vi "ge_TableFGV.vi"(4 "VKey":T1, 5 "Mod":bool, 6 "CtlRef":refnum<vi>, 7 "ge_TableCmnds":T7, 8 "error in":errorcluster, 9 "Cell Contents":T5, 10 "Specific Info":T4, 11 "ChanGrp.lvclass":refnum<class "ChanGrp.lvclass">) -> (0 "error out":errorcluster, 1 "Discard?":bool, 2 "ValIfDismissed":u16, 3 "ChanGrp.lvclass":refnum<class "ChanGrp.lvclass">)   [LabVIEW 2012]
uses:
  Custom Ctls Table/ge_TableCmnds.ctl
  Classes/Cfg Grandmaster/Class Chan Group/ChanGrp.lvclass
  Custom Ctls Table/ge_CellContents.ctl
  <vilib>/Utility/miscctls.llb/LVPoint32TypeDef.ctl
  Custom Ctls Table/ge_GrpSpecificInfo.ctl
  Common/Controls/TE_Designator.ctl
  <vilib>/event_ctls.llb/eventvkey.ctl
  Custom Ctrls/ge_FPCtrlRefLabel.ctl
  <vilib>/Utility/miscctls.llb/LVRowAndColumnTypeDef.ctl
  Custom Ctls Table/ge_StringVals.ctl
  Custom Ctls Table/ge_GlblCtrls.ctl
  <vilib>/Utility/miscctls.llb/LVRowAndColumnUnsignedTypeDef.ctl
  Custom Ctls Table/ge_HdrInfo.ctl
  Classes/Cfg Grandmaster/Class Chan Group/Read GrpName.vi
  Classes/Cfg Grandmaster/Class Chan Group/Read MeasType.vi
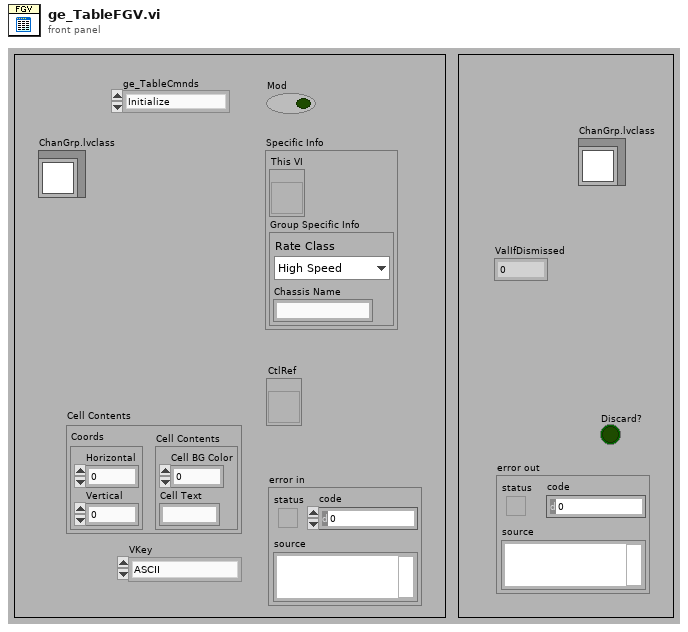
[diagram p1: front panel]
types:
  T1 = typedef "eventvkey.ctl" = enum16{"ASCII", "Enter", "Return", "Shift", "Ctrl", "Alt", "Cmd", "Opt", "Caps", "NumLock", "Clear", "Break", "Up", "Down", "Left", "Right", "Insert", "Delete", "Home", "End", "PageUp", "PageDown", "Escape", "Help", "Pause", "ScrollLock", "F1", "F2", "F3", "F4", "F5", "F6", "F7", "F8", "F9", "F10", "F11", "F12", "F13", "F14", "F15", "F16", "F17", "F18", "F19", "F20", "F21", "F22", "F23", "F24", "Play", "VolumeUp", "VolumeDown", "Mute", "Two Byte Char"}
  T2 = typedef "ge_GrpSpecificInfo.ctl" = cluster{"Rate Class":T3, "Chassis Name":string}
  T3 = typedef "TE_Designator.ctl" = enum16{"High Speed", "Low Speed"}
  T4 = cluster{"This VI":refnum<vi>, "Group Specific Info":T2}
  T5 = typedef "ge_CellContents.ctl" = cluster{"Cell Contents":cluster{"Cell Text":string, "Cell BG Color":u32}, "Coords":T6}
  T6 = typedef "LVPoint32TypeDef.ctl" = cluster{"Horizontal":i32, "Vertical":i32}
  T7 = typedef "ge_TableCmnds.ctl" = enum16{"Initialize", "Hide Cell Ctrls", "Position Ctrls", "Load Table", "Reset Table", "Clear Selections", "Ungchd Enter?", "Cell ValChng", "Click Ring", "Edit Cell", "Dismiss Menu", "Glbl Apply", "Calibrate", "Apply Settings", "Cell Key", "SaveChanList", "LoadChanDesc", "Shutdown"}
  T8 = typedef "LVRowAndColumnTypeDef.ctl" = cluster{"Row":i32, "Column":i32}
  T9 = typedef "ge_StringVals.ctl" = cluster{"String":string, "Value":u16}
  T10 = typedef "ge_GlblCtrls.ctl" = enum16{"Str0", "Bool0", "Bool1", "Int0", "Ring0", "Ring1", "Ring2", "Ring3", "Dbl0", "Dbl1", "Dbl2", "Dbl3", "Cal0", "Cal1", "Cal2", "None"}
  T11 = typedef "LVRowAndColumnUnsignedTypeDef.ctl" = cluster{"Row":u32, "Column":u32}
  T12 = typedef "ge_FPCtrlRefLabel.ctl" = cluster{"Label Array":string[], "Ref Array":refnum<vi>[]}
  T13 = typedef "DAQMan Definitions.ctl" = cluster{"Timing Engine Defs":variant, "Table Definitions":variant, "Ring Definitions":variant}
  T14 = typedef "ge_MeasType.ctl" = enum16{"Voltage", "Frequency", "Tachometer", "Dynamic", "Thermocouple", "RTD", "Strain", "Current", "Resistance"}
  T15 = typedef "ge_ColDef.ctl" = cluster{"ge_HdrNames":T16, "HdrInfo":T17}
  T16 = typedef "HeaderNames.ctl" = enum16{"Channel", "Device", "Spacer", "Description", "MB", "Range", "Terminal", "Coupling", "Thresh (V)", "Pulse/Rev", "Slope", "Min EU", "Min RPM", "mV/EU", "Iex", "Temp Units", "Type", "CJC Src", "CJC Val", "Ro", "Wire Cfg", "Strain Mode", "Vex", "Bridge Type", "GF", "Gauge Res", "Poisson", "Lead Res", "Init Strain", "GAF", "Scale", "Offset", "Unit (EU)", "dB?", "dB Ref", "Cal Mag", "Cal Units", "Max Temp", "Min Temp", "Max Strain", "Min Strain"}
  T17 = typedef "ge_HdrInfo.ctl" = cluster{"Hdr Width":i32, "Glbl Ctrl":T10}
  T18 = typedef "LVPositionTypeDef.ctl" = cluster{"Left":i32, "Top":i32}
  T19 = typedef "LVBoundsTypeDef.ctl" = cluster{"Width":u32, "Height":u32}
  T20 = cluster{"TopCtrlPos":T18, "CellSize":T19, "BtmCtrlPos":T18}
  T21 = typedef "LVRectTypeDef.ctl" = cluster{"Left":i16, "Top":i16, "Right":i16, "Bottom":i16}
  T22 = typedef "LVStringsAndValuesArrayTypeDef_U16.ctl" = cluster{"String":string, "Value":u16}[]
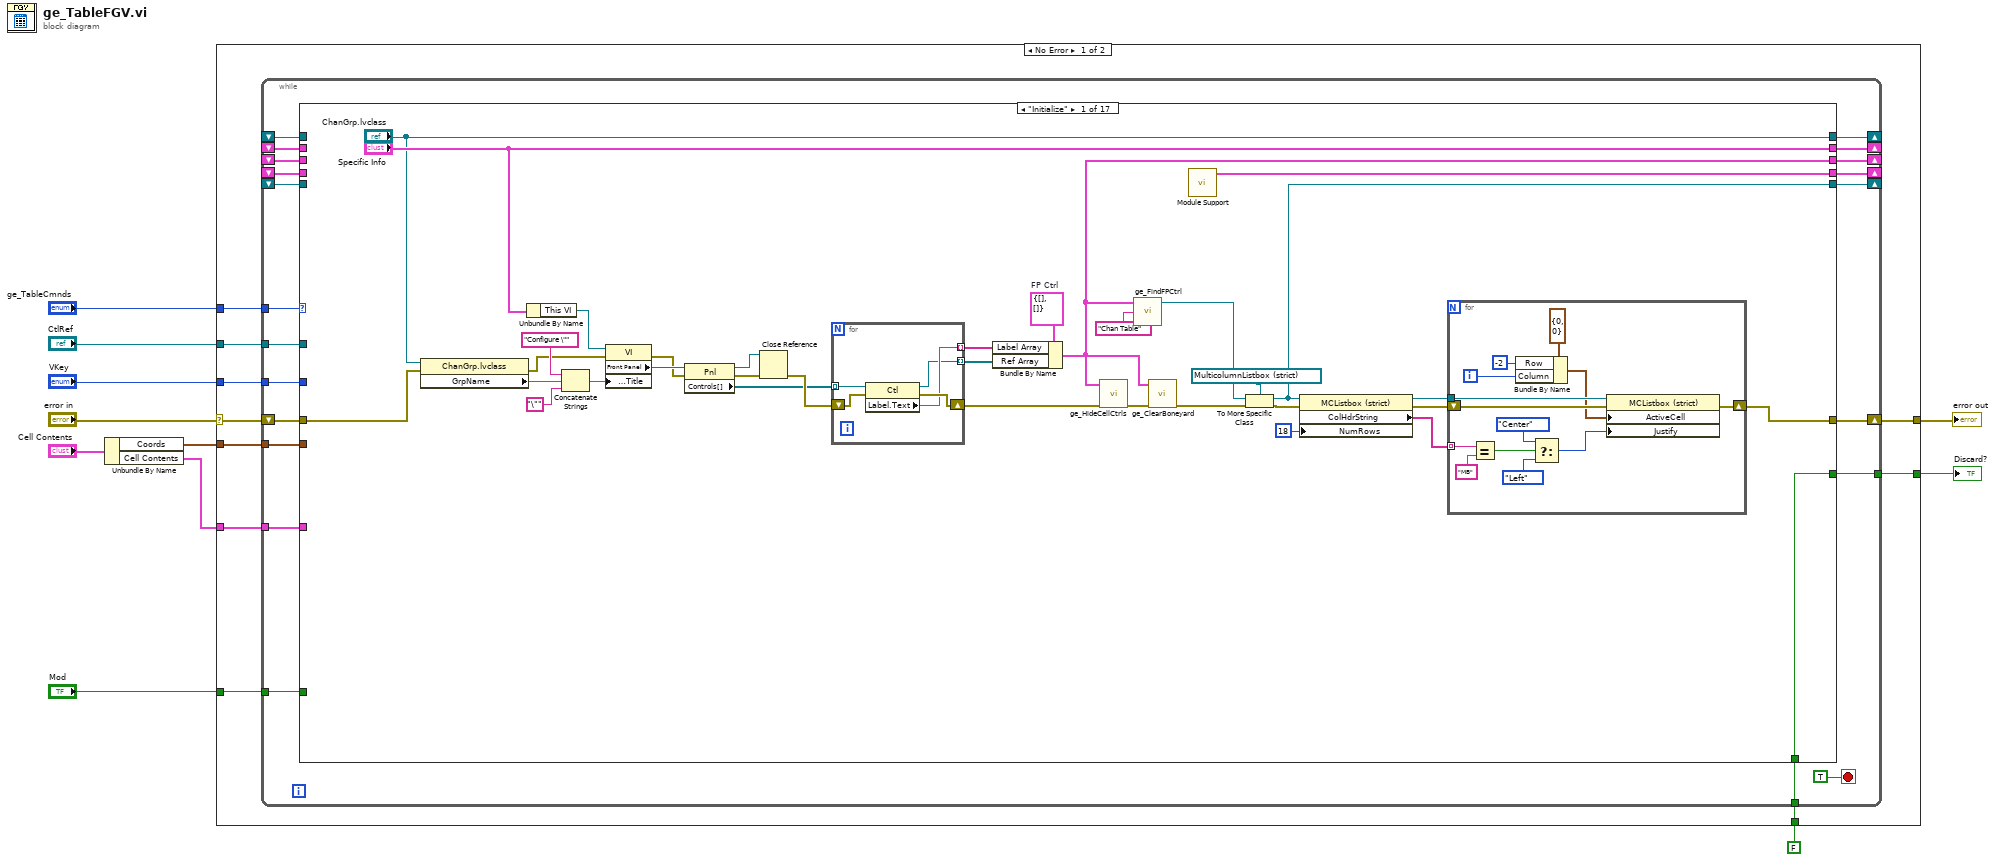
[diagram p0: block diagram]
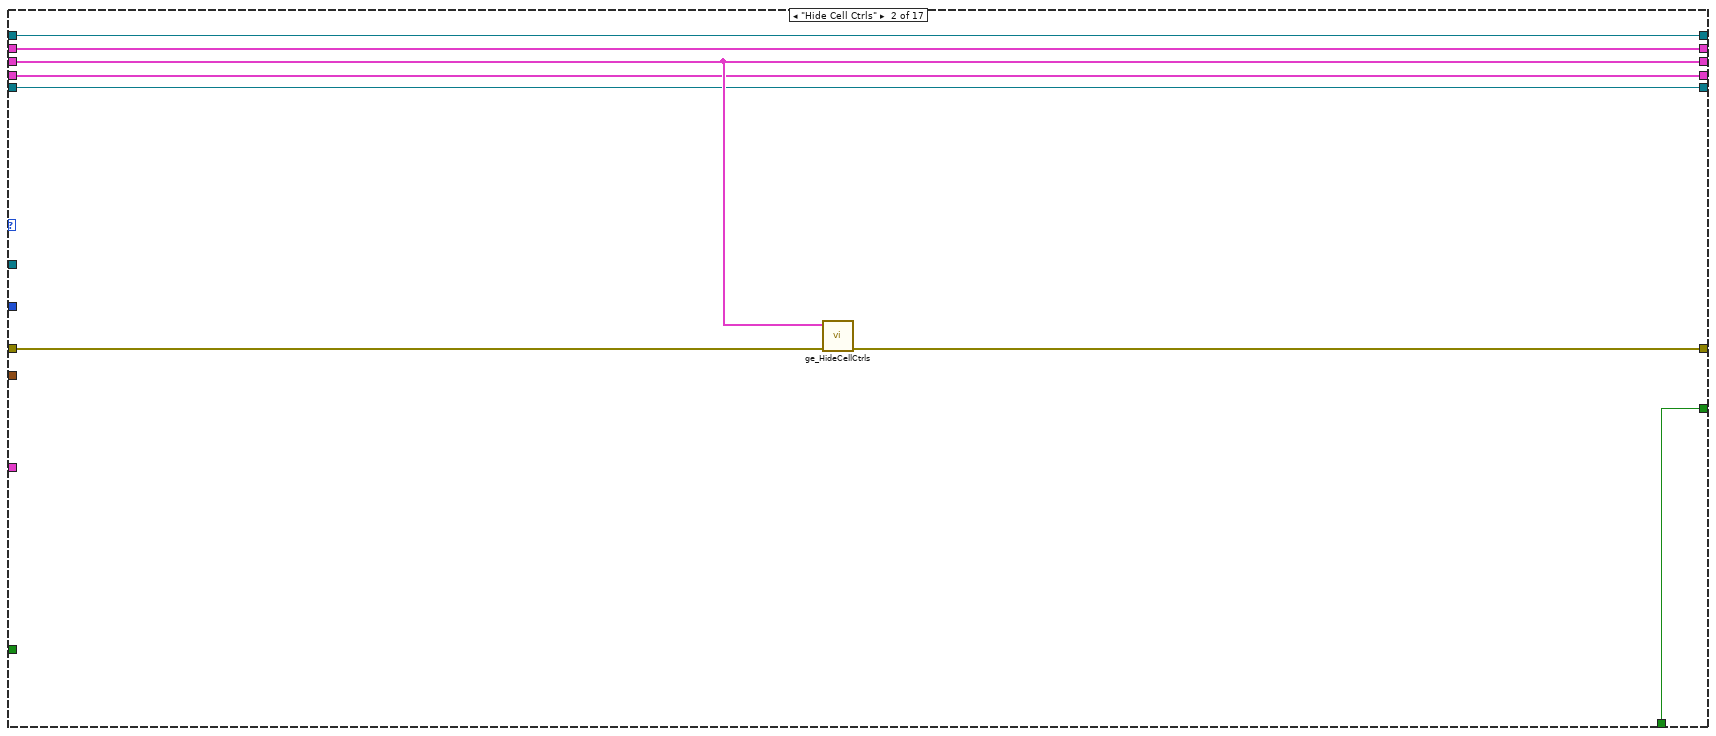
[diagram p2: hidden frame]
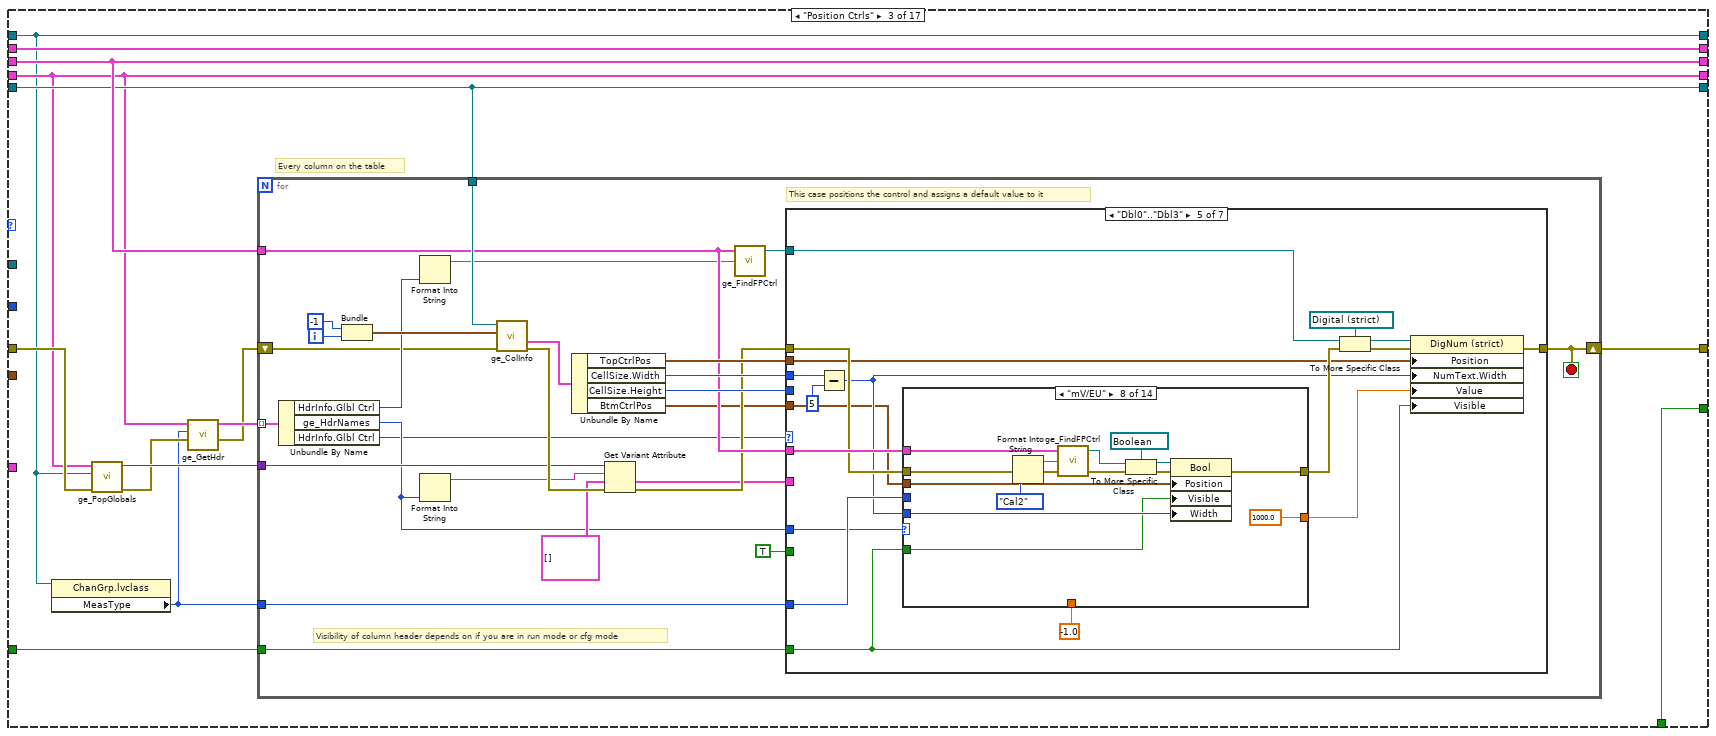
[diagram p3: hidden frame]
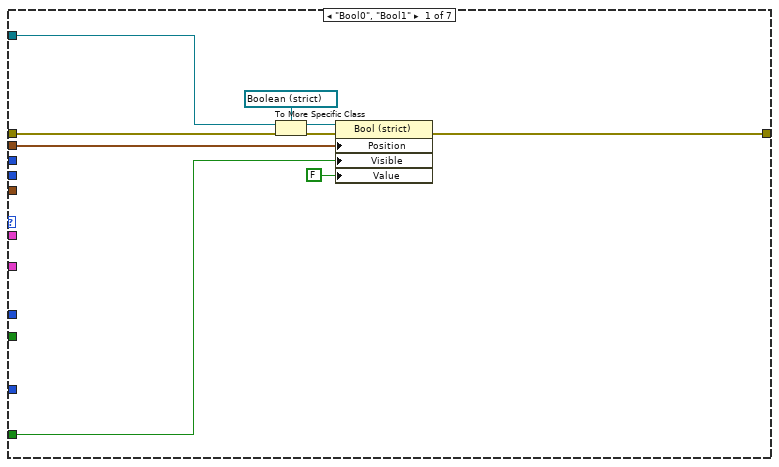
[diagram p4: hidden frame]
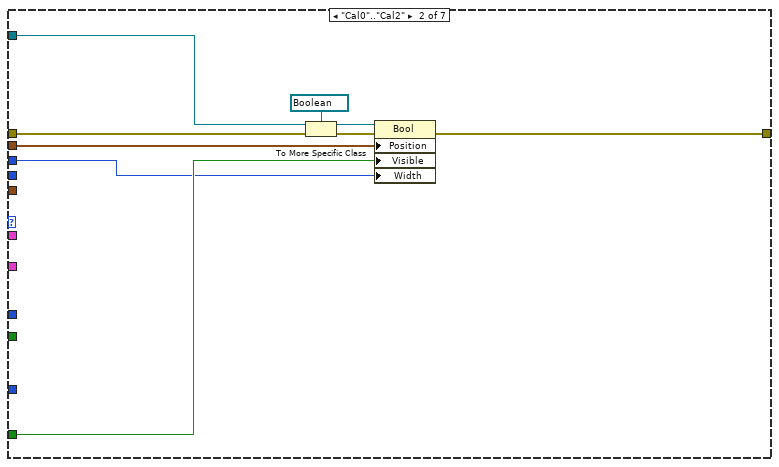
[diagram p5: hidden frame]
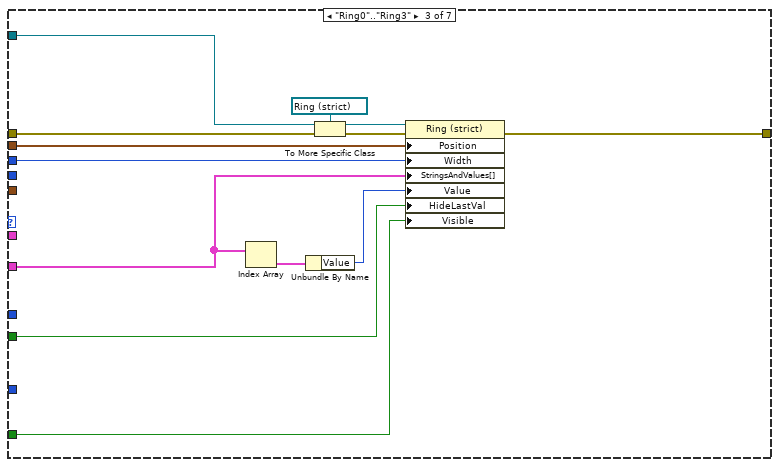
[diagram p6: hidden frame]
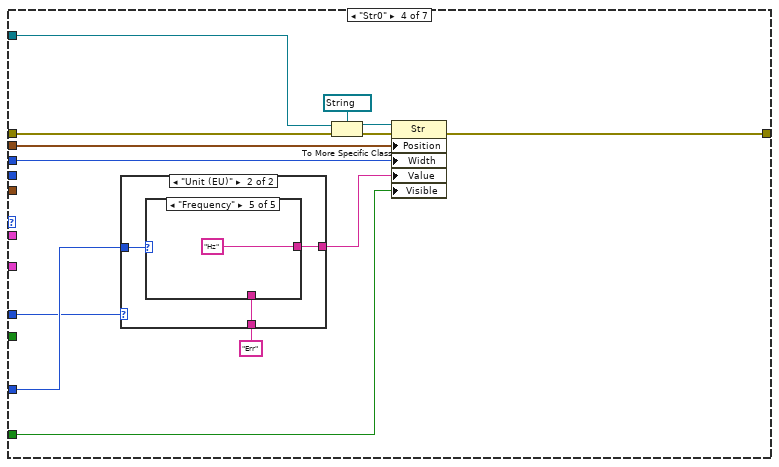
[diagram p7: hidden frame]
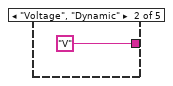
[diagram p10: hidden frame]
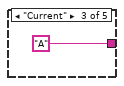
[diagram p11: hidden frame]
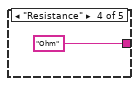
[diagram p12: hidden frame]
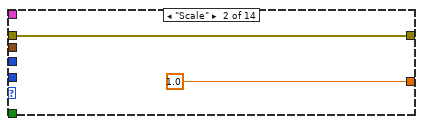
[diagram p14: hidden frame]
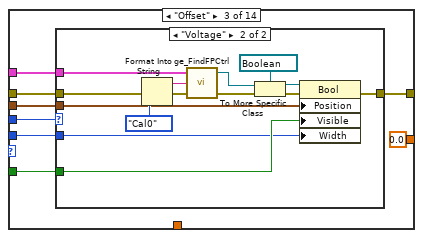
[diagram p15: hidden frame]
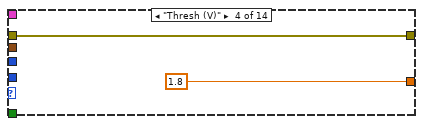
[diagram p17: hidden frame]
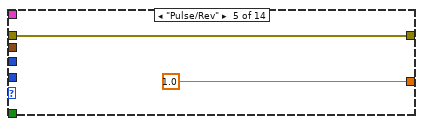
[diagram p18: hidden frame]
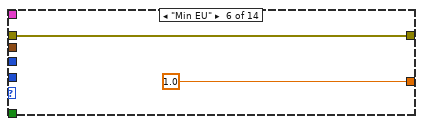
[diagram p19: hidden frame]
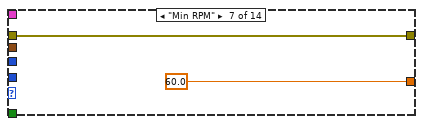
[diagram p20: hidden frame]
diagram:
  n1 = Unbundle By Name("Cell Contents") -> ("Coords"=w7:T6, "Cell Contents"=w6:cluster{"Cell Text":string, "Cell BG Color":u32})
  n2 = case shown="No Error" "error in" {
    selector: "error in" -> [w20 w1057]
    tunnel: [w21 w1057] -> w11
    tunnel: "ge_TableCmnds" -> [w19 _]
    tunnel: w7 -> [w18 _]
    tunnel: w6 -> [w17 _]
    tunnel: "CtlRef" -> [w16 _]
    tunnel: "Mod" -> [w15 _]
    tunnel: "VKey" -> [w14 _]
    tunnel: [w13 w1056] -> w3
    tunnel: FALSE ("Discard?") -> [w12 w1056]
    frame No Error {
      n3 = while {
        shift-right: [w42] -> w21
        shift-left: w20 -> [w41]
        shift-right: [w22] -> _
        shift-left: _ -> [w39]
        tunnel: w19 -> [w38]
        shift-right: [w37] -> _
        shift-left: _ -> [w36]
        tunnel: w18 -> [w35]
        tunnel: w17 -> [w34]
        shift-right: [w33] -> _
        shift-left: _ -> [w32]
        tunnel: w16 -> [w31]
        shift-right: [w30] -> _
        shift-left: _ -> [w29]
        tunnel: w15 -> [w28]
        tunnel: w14 -> [w27]
        tunnel: [w26] -> w13
        tunnel: w12 -> [w25]
        shift-right: [w24] -> _
        shift-left: _ -> [w23]
        stop <- TRUE stop-if-true
        n4 = case shown="\"Initialize\"" w38 {
          selector: w38 -> [_ _ _ w321 _ _ _ _ _ _ _ _ _ _ _ _ _]
          tunnel: [w51 w101 w110 w311 w352 w395 w468 w483 w513 w572 w709 w829 w874 w900 w966 w1039 w1046] -> w42
          tunnel: w41 -> [w45 w102 w111 w292 w343 w386 w465 w472 w508 w552 w713 w820 w867 w878 w962 w1034 w1055]
          tunnel: w39 -> [_ w95 w104 w294 w339 w382 w461 w476 w504 w551 w705 w799 w862 w880 w952 w1036 w1044]
          tunnel: [w48 w100 w115 w303 w356 w399 w466 w481 w509 w566 w710 w831 w865 w909 w970 w1043 w1047] -> w37
          tunnel: w36 -> [_ w100 w115 w303 w356 w399 w466 w481 w509 w566 w710 w831 w865 w909 w970 w1043 w1047]
          tunnel: w35 -> [_ _ _ _ _ _ _ w487 _ _ _ _ _ _ _ _ _]
          tunnel: w34 -> [_ _ _ _ _ _ _ _ _ _ _ _ _ _ _ _ _]
          tunnel: ["Specific Info" w99 w116 w301 w357 w400 w467 w482 w511 w565 w712 w833 w873 w901 w968 w1042 w1053] -> w33
          tunnel: w32 -> [_ w99 w116 w301 w357 w400 w467 w482 w511 w565 w712 w833 w873 w901 w968 w1042 w1053]
          tunnel: w31 -> [_ _ _ _ _ _ _ _ w510 w559 w714 w830 _ w898 w961 _ _]
          tunnel: [w56 w98 w113 w302 w353 w396 w464 w480 w507 w567 w711 w832 w872 w889 w954 w1041 w1054] -> w30
          tunnel: w29 -> [_ w98 w113 w302 w354 w397 w464 w480 w507 w567 w711 w832 w872 w889 w954 w1041 w1054]
          tunnel: w28 -> [_ _ w114 _ _ _ _ w479 _ _ _ _ _ _ _ _ _]
          tunnel: w27 -> [_ _ _ _ _ _ _ _ _ w571 w707 _ _ _ _ _ _]
          tunnel: [w53 w97 w112 w299 w355 w398 w463 w478 w506 w568 w708 w828 w864 w887 w959 w1040 w1051] -> w26
          tunnel: w25 -> [w53 w97 w112 w299 w355 w398 w463 _ w506 _ w708 w828 w864 w887 w959 w1040 w1051]
          tunnel: [w47 w96 w105 w298 w340 w383 w462 w477 w505 w555 w706 w802 w863 w885 w953 w1037 w1045] -> w24
          tunnel: w23 -> [_ w96 w105 w298 w340 w383 w462 w477 w505 w555 w706 w802 w863 w885 w953 w1037 w1045]
          tunnel: ["ChanGrp.lvclass" w95 w104 w294 w339 w382 w461 w476 w504 w551 w705 w799 w862 w880 w952 w1035 w1044] -> w22
          frame "Initialize" {
            w71 = T12 {"Label Array"=[], "Ref Array"=[]}  # FP Ctrl
            n5 = property class="ChanGrp.lvclass"(reference="ChanGrp.lvclass", error in=w45) -> (error out=w44:errorcluster, "GrpName"=w46:string)  [unwired: 1 out]
            n6 = Unbundle By Name("Specific Info") -> ("This VI"=w54:refnum<vi>)
            n7 = Concatenate Strings("Configure \"" ("string"), w46, "\"") -> (w62:string)
            n8 = property class="VI"(reference=w54, error in=w44, "Front Panel.Title"=w62) -> (error out=w65:errorcluster, "Front Panel"=w66:refnum<vi>)  [unwired: 1 out]
            n9 = property class="Pnl"(reference=w66, error in=w65) -> (reference out=w70:refnum<vi>, error out=w68:errorcluster, "Controls[]"=w67:refnum<vi>[])
            n10 = Close Reference(reference=w70, error in (no error)=w68) -> (error out=w69:errorcluster)
            n11 = for {
              tunnel: w67 -> [w81] mode=indexing
              shift-right: [w79] -> w64
              shift-left: w69 -> [w80]
              tunnel: [w78] -> w58 mode=indexing
              tunnel: [w77] -> w57 mode=indexing
              n12 = property class="Ctl"(reference=w81, error in=w80) -> (reference out=w77:refnum<vi>, error out=w79:errorcluster, "Label.Text"=w78:string)
            }
            n13 = Bundle By Name(cluster=w71, "Label Array"=w58, "Ref Array"=w57) -> (w48:T12)
            n14 = call "ge_HideCellCtrls.vi"("error IO"=w64, "FP Ctrl"=w48) -> ("error out"=w50:errorcluster)  [unwired: 9 in]
            n15 = call "ge_FindFPCtrl.vi"("Ctrl Name"="Chan Table" ("Name"), "FP Ctrl"=w48) -> ("Ctrl Ref"=w59:refnum<vi>)  [unwired: 3 in]
            n16 = call "ge_ClearBoneyard.vi"("error in"=w50, "FP Ctrl"=w48) -> ("error out"=w49:errorcluster)  [unwired: 9 in]
            n17 = call "Module Support.vi"() -> ("ge_DAQManDefinitions"=w47:T13)  [unwired: 9 in]
            n18 = To More Specific Class(target class=refnum<vi> refnum ("reference"), reference=w59, error in=w49) -> (specific class reference=w56:refnum<vi>, error out=w60:errorcluster)
            n19 = property class="MCListbox (strict)"(reference=w56, error in=w60, "NumRows"=u32 18 ("Number of Rows")) -> (reference out=w73:refnum<vi>, error out=w74:errorcluster, "ColHdrString"=w72:string[])
            n20 = for {
              tunnel: w73 -> [w93]
              shift-right: [w89] -> w51
              shift-left: w74 -> [w94]
              tunnel: w72 -> [w88] mode=indexing
              i -> [w85]
              n21 = Equal?(x=w88, y="MB" ("element")) -> (x = y?=w86:bool)
              n22 = Bundle By Name(cluster=T8 {"Row"=0, "Column"=0} ("Active Cell:Active Cell"), "Row"=-2, "Column"=w85) -> (w90:T8)
              n23 = Select(t=enum16{"Left", "Center", "Right"}."Center" ("Active Cell:Cell Justification"), s=w86, f=enum16{"Left", "Center", "Right"}."Left" ("Active Cell:Cell Justification")) -> (s? t:f=w82:enum16{"Left", "Center", "Right"})
              n24 = property class="MCListbox (strict)"(reference=w93, error in=w94, "ActiveCell"=w90, "Justify"=w82) -> (error out=w89:errorcluster)  [unwired: 1 out]
            }
          }
          frame "Hide Cell Ctrls" {
            n25 = call "ge_HideCellCtrls.vi"("error IO"=w102, "FP Ctrl"=w100) -> ("error out"=w101:errorcluster)  [unwired: 9 in]
          }
          frame "Position Ctrls" {
            # "Every column on the table"
            n26 = property class="ChanGrp.lvclass"(reference=w104) -> ("MeasType"=w103:T14)  [unwired: 1 in, 2 out]
            n27 = call "ge_PopGlobals.vi"("error in"=w111, "ChanGrp.lvclass"=w104, "ge_DAQManDefinitions"=w105) -> ("error out"=w107:errorcluster, "Ring Support For Group"=w109:variant)  [unwired: 6 in, 1 out]
            n28 = call "ge_GetHdr.vi"("error in"=w107, "MeasType"=w103, "ge_DAQManDefinitions"=w105) -> ("error out"=w106:errorcluster, "Table Hdrs"=w108:T15[])  [unwired: 7 in]
            n29 = for {
              tunnel: w108 -> [w138] mode=indexing
              tunnel: w114 -> [w137]
              tunnel: w115 -> [w130]
              tunnel: w113 -> [w132]
              tunnel: w103 -> [w131]
              shift-right: [w127] -> w110
              shift-left: w106 -> [w121]
              tunnel: w109 -> [w123]
              i -> [w135]
              stop <- w127 stop-if-true
              # "This case positions the control and assigns a default value to it"
              # "Visibility of column header depends on if you are in run mode or cfg mode"
              n30 = Unbundle By Name(w138) -> ("HdrInfo.Glbl Ctrl"=w129:T10, "ge_HdrNames"=w120:T16, "HdrInfo.Glbl Ctrl"=w119:T10)
              n31 = Bundle("Column"=-1, w135) -> (w133:cluster{"Column":i32, i32})  [unwired: 1 in]
              n32 = Format Into String(w129) -> (resulting string=w128:string)  [unwired: 3 in, 1 out]
              n33 = Format Into String(w120) -> (resulting string=w117:string)  [unwired: 3 in, 1 out]
              n34 = call "ge_ColInfo.vi"("error in"=w121, "Active Cell"=w133, "Table Ref"=w132) -> ("error out"=w126:errorcluster, "Ctrl Size Pos"=w143:T20)  [unwired: 7 in]
              n35 = Unbundle By Name(w143) -> ("TopCtrlPos"=w142:T18, "CellSize.Width"=w141:u32, "CellSize.Height"=w140:u32, "BtmCtrlPos"=w118:T18)
              n36 = Get Variant Attribute(Variant=w123, name=w117, default value (empty Variant)=T9[] [] ("String and Values"), error in=w126) -> (value=w122:T9[], error out=w125:errorcluster)  [unwired: 2 out]
              n37 = call "ge_FindFPCtrl.vi"("Ctrl Name"=w128, "FP Ctrl"=w130) -> ("Ctrl Ref"=w134:refnum<vi>)  [unwired: 3 in]
              n38 = case shown="\"Dbl0\"..\"Dbl3\"" w119 {
                tunnel: w125 -> [w149 w158 w167 w184 w201 w281 w290]
                tunnel: w142 -> [w152 w161 w173 w181 w200 w279 _]
                tunnel: w141 -> [_ w156 w171 w180 w207 w278 _]
                tunnel: w140 -> [_ _ _ _ _ _ _]
                tunnel: TRUE ("Hide Last Value") -> [_ _ w172 _ _ _ _]
                tunnel: [w150 w159 w174 w182 w210 w282 w290] -> w127
                tunnel: w137 -> [w151 w160 w168 w179 w206 w277 _]
                tunnel: w134 -> [w148 w157 w163 w183 w205 w280 _]
                tunnel: w131 -> [_ _ _ w178 w203 _ _]
                tunnel: w130 -> [_ _ _ _ w204 _ _]
                tunnel: w122 -> [_ _ w162 _ _ _ _]
                tunnel: w120 -> [_ _ _ w176 w198 w276 _]
                tunnel: w118 -> [_ _ _ _ w197 _ _]
                frame "Bool0", "Bool1" {
                  n39 = To More Specific Class(target class=refnum<vi> refnum ("Bool0"), reference=w148, error in=w149) -> (specific class reference=w147:refnum<vi>, error out=w146:errorcluster)
                  n40 = property on="Property Node" class="Bool (strict)"(reference=w147, error in=w146, "Position"=w152, "Visible"=w151, "Value"=FALSE) -> (error out=w150:errorcluster)  [unwired: 1 out]
                }
                frame "Cal0".."Cal2" {
                  n41 = To More Specific Class(target class=refnum<vi> refnum ("Cal0"), reference=w157, error in=w158) -> (specific class reference=w153:refnum<vi>, error out=w154:errorcluster)
                  n42 = property on="Property Node" class="Bool"(reference=w153, error in=w154, "Position"=w161, "Visible"=w160, "Width"=w156) -> (error out=w159:errorcluster)  [unwired: 1 out]
                }
                frame "Ring0".."Ring3" {
                  n43 = Index Array(array=w162) -> (element=w170:T9)  [unwired: 1 in]
                  n44 = Unbundle By Name(w170) -> ("Value"=w169:u16)
                  n45 = To More Specific Class(target class=refnum<vi> refnum ("reference"), reference=w163, error in=w167) -> (specific class reference=w164:refnum<vi>, error out=w166:errorcluster)
                  n46 = property on="Property Node" class="Ring (strict)"(reference=w164, error in=w166, "Position"=w173, "Width"=w171, "StringsAndValues[]"=w162, "Value"=w169, "HideLastVal"=w172, "Visible"=w168) -> (error out=w174:errorcluster)  [unwired: 1 out]
                }
                frame "Str0" {
                  n47 = case shown="\"Unit (EU)\"" w176 {
                    tunnel: w178 -> [_ w191]
                    tunnel: [w188 w190] -> w177
                    tunnel: "Err" ("EU") -> [w188 w189]
                    frame Default {
                    }
                    frame "Unit (EU)" {
                      n48 = case shown="\"Frequency\"" w191 {
                        tunnel: [w192 "V" ("EU") "A" ("EU") "Ohm" ("EU") "Hz" ("EU")] -> w190
                        tunnel: w189 -> [w192 _ _ _ _]
                        frame Default {
                        }
                        frame "Voltage", "Dynamic" {
                        }
                        frame "Current" {
                        }
                        frame "Resistance" {
                        }
                        frame "Frequency" {
                        }
                      }
                    }
                  }
                  n49 = To More Specific Class(target class=refnum<vi> refnum ("reference"), reference=w183, error in=w184) -> (specific class reference=w186:refnum<vi>, error out=w185:errorcluster)
                  n50 = property on="Property Node" class="Str"(reference=w186, error in=w185, "Position"=w181, "Width"=w180, "Value"=w177, "Visible"=w179) -> (error out=w182:errorcluster)  [unwired: 1 out]
                }
                frame "Dbl0".."Dbl3" {
                  n51 = Subtract(x=w207, y=u32 5) -> (x-y=w199:u32)
                  n52 = case shown="\"mV/EU\"" w198 {
                    tunnel: [w216 1.0 ("Value") 0.0 ("Value") 1.8 ("Value") 1.0 ("Value") 1.0 ("Value") 60.0 ("Value") 1000.0 ("Value") 1.0 ("Value") 1.0 ("Value") 25.0 ("Value") 2.0 ("Value") 0.3 ("Value") 0.0 ("Value")] -> w209
                    tunnel: -1.0 ("Value") -> [w216 _ _ _ _ _ _ _ _ _ _ _ _ _]
                    tunnel: w206 -> [_ _ w225 _ _ _ _ w250 _ _ _ _ _ _]
                    tunnel: w204 -> [_ _ w224 _ _ _ _ w254 _ _ _ _ _ _]
                    tunnel: w203 -> [_ _ w223 _ _ _ _ _ _ _ _ _ _ _]
                    tunnel: [w215 w217 w222 w242 w244 w246 w248 w249 w264 w266 w268 w270 w272 w274] -> w202
                    tunnel: w201 -> [w215 w217 w221 w242 w244 w246 w248 w253 w264 w266 w268 w270 w272 w274]
                    tunnel: w197 -> [_ _ w220 _ _ _ _ w252 _ _ _ _ _ _]
                    tunnel: w199 -> [_ _ w219 _ _ _ _ w251 _ _ _ _ _ _]
                    frame Default {
                    }
                    frame "Scale" {
                    }
                    frame "Offset" {
                      n53 = case shown="\"Voltage\"" w223 {
                        tunnel: w225 -> [_ w234]
                        tunnel: w224 -> [_ w233]
                        tunnel: [w227 w232] -> w222
                        tunnel: w220 -> [_ w231]
                        tunnel: w221 -> [w227 w230]
                        tunnel: w219 -> [_ w228]
                        frame Default {
                        }
                        frame "Voltage" {
                          n54 = Format Into String(error in=w230, ge_GlblCtrls."Cal0" ("Glbl Ctrl")) -> (resulting string=w240:string, error out=w229:errorcluster)  [unwired: 2 in]
                          n55 = call "ge_FindFPCtrl.vi"("Ctrl Name"=w240, "FP Ctrl"=w233) -> ("Ctrl Ref"=w238:refnum<vi>)  [unwired: 3 in]
                          n56 = To More Specific Class(target class=refnum<vi> refnum ("Cal0"), reference=w238, error in=w229) -> (specific class reference=w236:refnum<vi>, error out=w235:errorcluster)
                          n57 = property on="Property Node" class="Bool"(reference=w236, error in=w235, "Position"=w231, "Visible"=w234, "Width"=w228) -> (error out=w232:errorcluster)  [unwired: 1 out]
                        }
                      }
                    }
                    frame "Thresh (V)" {
                    }
                    frame "Pulse/Rev" {
                    }
                    frame "Min EU" {
                    }
                    frame "Min RPM" {
                    }
                    frame "mV/EU" {
                      n58 = Format Into String(error in=w253, ge_GlblCtrls."Cal2" ("Glbl Ctrl")) -> (resulting string=w261:string, error out=w255:errorcluster)  [unwired: 2 in]
                      n59 = call "ge_FindFPCtrl.vi"("Ctrl Name"=w261, "FP Ctrl"=w254) -> ("Ctrl Ref"=w259:refnum<vi>)  [unwired: 3 in]
                      n60 = To More Specific Class(target class=refnum<vi> refnum ("Cal0"), reference=w259, error in=w255) -> (specific class reference=w257:refnum<vi>, error out=w256:errorcluster)
                      n61 = property on="Property Node" class="Bool"(reference=w257, error in=w256, "Position"=w252, "Visible"=w250, "Width"=w251) -> (error out=w249:errorcluster)  [unwired: 1 out]
                    }
                    frame "dB Ref" {
                    }
                    frame "Cal Mag" {
                    }
                    frame "CJC Val" {
                    }
                    frame "GF" {
                    }
                    frame "Poisson" {
                    }
                    frame "Lead Res" {
                    }
                  }
                  n62 = To More Specific Class(target class=refnum<vi> refnum ("reference"), reference=w205, error in=w202) -> (specific class reference=w211:refnum<vi>, error out=w212:errorcluster)
                  n63 = property on="Property Node" class="DigNum (strict)"(reference=w211, error in=w212, "Position"=w200, "NumText.Width"=w199, "Value"=w209, "Visible"=w206) -> (error out=w210:errorcluster)  [unwired: 1 out]
                }
                frame "Int0" {
                  n64 = case shown="\"Gauge Res\"" w276 {
                    tunnel: [0 ("Value") 350 ("Value")] -> w275
                    frame Default {
                    }
                    frame "Gauge Res" {
                    }
                  }
                  n65 = Subtract(x=w278, y=u32 5) -> (x-y=w284:u32)
                  n66 = To More Specific Class(target class=refnum<vi> refnum ("reference"), reference=w280, error in=w281) -> (specific class reference=w285:refnum<vi>, error out=w286:errorcluster)
                  n67 = property on="Property Node" class="DigNum (strict)"(reference=w285, error in=w286, "Position"=w279, "NumText.Width"=w284, "Value"=w275, "Visible"=w277) -> (error out=w282:errorcluster)  [unwired: 1 out]
                }
                frame "None" {
                }
              }
            }
          }
          frame "Load Table", "Reset Table" {
            n68 = property class="ChanGrp.lvclass"(reference=w294, error in=w292) -> (error out=w291:errorcluster, "MeasType"=w293:T14)  [unwired: 1 out]
            n69 = call "ge_GetHdrInfo.vi"("ge_DAQManDefinitions"=w298, "MeasType"=w293) -> ("Hdr Widths"=w297:i32[], "Hdr Name"=w295:T16[])  [unwired: 7 in, 1 out]
            n70 = for {
              tunnel: w295 -> [w327] mode=indexing
              tunnel: [w326] -> w296 mode=indexing
              n71 = Format Into String(w327) -> (resulting string=w326:string)  [unwired: 3 in, 1 out]
            }
            n72 = call "CellColors.vi"() -> ("Normal"=w324:u32)  [unwired: 8 in, 3 out]
            n73 = Add Array Elements(numeric array=w297) -> (sum=w306:i32)
            n74 = Add(x=u32 25, y=w306) -> (x+y=w315:u32)
            n75 = property on="Property Node" class="MCListbox (strict)"(reference=w302, error in=w291, "Value"=i32[] [], "ActiveCell"=T8 {"Row"=-2, "Column"=-2} ("Active Cell:Active Cell"), "CellBG"=w324, "TopLeft"=T11 {"Row"=0, "Column"=0} ("Top Left Visible Cell"), "ColHdrString"=w296, "Width"=w315) -> (reference out=w320:refnum<vi>, error out=w319:errorcluster)
            n76 = for {
              shift-right: [w333] -> w317
              shift-left: w320 -> [w335]
              shift-right: [w332] -> w318
              shift-left: w319 -> [w334]
              tunnel: w297 -> [w331] mode=indexing
              i -> [w330]
              n77 = Bundle(-2, w330) -> (w328:cluster{i32, i32})  [unwired: 1 in]
              n78 = property on="Property Node" class="MCListbox (strict)"(reference=w335, error in=w334, "ActiveCell"=w328, "Width"=w331) -> (reference out=w333:refnum<vi>, error out=w332:errorcluster)
            }
            n79 = Unbundle By Name(w301) -> ("This VI"=w300:refnum<vi>, "Group Specific Info.Rate Class"=w304:T3)
            n80 = call "ge_TableDefaults.vi"("Timing Engine"=w304, "ge_TableCmnds"=w321, "error in"=w318, "ge_DAQManDefinitions"=w298, "ChanGrp.lvclass"=w294, "Chan Table"=w317) -> ("error out"=w314:errorcluster)  [unwired: 4 in, 1 out]
            n81 = property class="VI"(reference=w300, error in=w314) -> (reference out=w313:refnum<vi>, error out=w312:errorcluster, "Front Panel.PanelBounds"=w310:T21)
            n82 = Unbundle By Name(w310) -> ("Left"=w308:i16)
            n83 = Compound Arithmetic op=ADD(w308, w306, 60 ("value")) -> (w307:i32)
            n84 = Bundle By Name(cluster=w310, "Right"=w307) -> (w309:T21)
            n85 = property class="VI"(reference=w313, error in=w312, "Front Panel.PanelBounds"=w309) -> (error out=w311:errorcluster)  [unwired: 1 out]
          }
          frame "SaveChanList" {
            n86 = call <vilib>:"Application Directory.vi"() -> ("Application Directory"=w349:path)
            n87 = Build Path(base path=w349, name or relative path="Channel Descriptions") -> (appended path=w351:path)
            n88 = call <vilib>:"Check if File or Folder Exists.vi"("error in (no error)"=w343, "path"=w351) -> ("error out"=w346:errorcluster, "file or folder exists?"=w345:bool, "dup path"=w344:path)  [unwired: 7 in]
            n89 = case shown="False" w345 {
              tunnel: w344 -> [w376 w377]
              tunnel: w346 -> [w375 w378]
              tunnel: [w374 w378] -> w337
              tunnel: [w373 w377] -> w347
              frame False {
                n90 = Create Folder(path (use dialog)=w376, error in=w375) -> (created path=w373:path, error out=w374:errorcluster)  [unwired: 1 in, 1 out]
              }
              frame True {
              }
            }
            n91 = property class="ChanGrp.lvclass"(reference=w339, error in=w337) -> (error out=w336:errorcluster, "GrpName"=w338:string)  [unwired: 1 out]
            n92 = call "File Dialog"("start path"=w347, "default name"=w338, "error in"=w336, "pattern (all files)"="*.csv") -> ("selected path"=w341:path, "error out"=w342:errorcluster)  [unwired: 8 in, 2 out]
            n93 = case shown="No Error" w342 {
              selector: w342 -> [w361 w371]
              tunnel: w354 -> [w368 w372]
              tunnel: [w367 w372] -> w353
              tunnel: [w362 w370] -> w352
              tunnel: w341 -> [w360 _]
              frame No Error {
                n94 = property on="Property Node" class="MCListbox (strict)"(reference=w368, error in=w361) -> (reference out=w367:refnum<vi>, error out=w366:errorcluster, "ItemNames"=w365:string[][])
                n95 = Array Subset(array=w365, index (col)=0 ("index"), length (col)=4 ("length")) -> (w358:string[][])  [unwired: 2 in]
                n96 = call "DAQMan Write To Spreadsheet File (String).vi"("delimiter (\\t)"="," ("delimiter (\\t)"), "error in"=w366, "2D data"=w358, "file path (dialog if empty)"=w360) -> ("error out"=w362:errorcluster)  [unwired: 6 in, 1 out]
              }
              frame Error {
                # "Cancel Button"
                n97 = call "DAQMan Clear Specific Error.vi"("error in"=w371, "code"=43) -> ("error out"=w370:errorcluster)  [unwired: 9 in]
              }
            }
          }
          frame "LoadChanDesc" {
            n98 = call <vilib>:"Application Directory.vi"() -> ("Application Directory"=w392:path)
            n99 = Build Path(base path=w392, name or relative path="Channel Descriptions") -> (appended path=w394:path)
            n100 = call <vilib>:"Check if File or Folder Exists.vi"("error in (no error)"=w386, "path"=w394) -> ("error out"=w389:errorcluster, "file or folder exists?"=w388:bool, "dup path"=w387:path)  [unwired: 7 in]
            n101 = case shown="False" w388 {
              tunnel: w387 -> [w458 w459]
              tunnel: w389 -> [w457 w460]
              tunnel: [w456 w460] -> w380
              tunnel: [w455 w459] -> w390
              frame False {
                n102 = Create Folder(path (use dialog)=w458, error in=w457) -> (created path=w455:path, error out=w456:errorcluster)  [unwired: 1 in, 1 out]
              }
              frame True {
              }
            }
            n103 = property class="ChanGrp.lvclass"(reference=w382, error in=w380) -> (error out=w379:errorcluster, "GrpName"=w381:string)  [unwired: 1 out]
            n104 = call "File Dialog2"("start path"=w390, "default name"=w381, "error in"=w379, "pattern (all files)"="*.csv") -> ("selected path"=w384:path, "error out"=w385:errorcluster)  [unwired: 8 in, 2 out]
            n105 = case shown="No Error" w385 {
              selector: w385 -> [w422 w453]
              tunnel: w397 -> [w423 w454]
              tunnel: [w419 w454] -> w396
              tunnel: [w418 w452] -> w395
              tunnel: w384 -> [w420 _]
              frame No Error {
                n106 = call "DAQMan Read From Spreadsheet File (string).vi"("file path (dialog if empty)"=w420, "error in"=w422, "delimiter (\\t)"="," ("delimiter (\\t)")) -> ("all rows"=w408:string[][], "error out"=w421:errorcluster)  [unwired: 7 in, 4 out]
                n107 = property on="Property Node" class="MCListbox (strict)"(reference=w423, error in=w421) -> (reference out=w414:refnum<vi>, error out=w412:errorcluster, "ItemNames"=w410:string[][])
                n108 = Index Array(array=w410, index (col)=0 ("disabled index (col)")) -> (element=w417:string[])  [unwired: 1 in]
                n109 = Index Array(array=w408, index (col)=0 ("disabled index (col)")) -> (element=w416:string[])  [unwired: 1 in]
                n110 = for {
                  tunnel: w417 -> [w434] mode=indexing
                  tunnel: w416 -> [w435]
                  shift-right: [w426] -> w415
                  shift-left: w410 -> [w427]
                  shift-right: [w430] -> w413
                  shift-left: w414 -> [w431]
                  shift-right: [w428] -> w411
                  shift-left: w412 -> [w429]
                  tunnel: w408 -> [w433]
                  shift-right: [w424] -> w405
                  shift-left: 0 -> [w425]
                  n111 = Search 1D Array(1D array=w435, element=w434) -> (index of element=w432:i32)  [unwired: 1 in]
                  n112 = case shown="Default" w432 {
                    selector: w432 -> [_ w444]
                    tunnel: w433 -> [_ w450]
                    tunnel: w431 -> [w439 w449]
                    tunnel: [w439 w449] -> w430
                    tunnel: w429 -> [w438 w448]
                    tunnel: [w438 w448] -> w428
                    tunnel: w427 -> [w437 w446]
                    tunnel: [w437 w445] -> w426
                    tunnel: w425 -> [w436 w442]
                    tunnel: [w436 w441] -> w424
                    frame -1 {
                    }
                    frame Default {
                      w440 = 3 ("index")
                      n113 = Index Array(array=w450, index (row)=w444) -> (element=w447:string[])  [unwired: 1 in]
                      n114 = Index Array(array=w447, index=w440) -> (element=w443:string)
                      n115 = Increment(x=w442) -> (x+1=w441:i32)
                      n116 = Replace Array Subset(array=w446, new element=w443, index (row)=w444, index (col)=w440) -> (w445:string[][])
                    }
                  }
                }
                n117 = Number To Decimal String(number=w405) -> (decimal integer string=w404:string)  [unwired: 1 in]
                n118 = property on="Property Node" class="MCListbox (strict)"(reference=w413, error in=w411, "ItemNames"=w415) -> (reference out=w419:refnum<vi>, error out=w418:errorcluster)
                n119 = Concatenate Strings(w404, " channel descriptions imported." ("string")) -> (w402:string)
                n120 = One Button Dialog(message=w402) -> ()  [unwired: 1 in, 1 out]
              }
              frame Error {
                # "Cancel Button"
                n121 = call "DAQMan Clear Specific Error.vi"("error in"=w453, "code"=43) -> ("error out"=w452:errorcluster)  [unwired: 9 in]
              }
            }
          }
          frame "Clear Selections" {
            n122 = property on="Property Node" class="MCListbox (strict)"(reference=w464, error in=w465, "Value"=i32[] [] ("CfgTable")) -> (error out=w468:errorcluster)  [unwired: 1 out]
          }
          frame "Edit Cell" {
            n123 = property class="ChanGrp.lvclass"(reference=w476, error in=w472) -> (reference out=w475:refnum<class "ChanGrp.lvclass">, error out=w473:errorcluster, "MeasType"=w474:T14)
            n124 = call "GetChanContents.vi"("error in"=w473, "ChanGrp.lvclass"=w475) -> ("error out"=w470:errorcluster, "Num of Chans"=w471:i32)  [unwired: 3 in, 5 out]
            n125 = invoke class="MCListbox (strict)" method="Point To Row Column"(reference=w480, error in=w470, "Point"=w487) -> (error out=w484:errorcluster, "InBounds"=w489:bool, "CellPosition"=w488:T8)  [unwired: 4 in, 4 out]
            n126 = Unbundle By Name(w488) -> ("Row"=w491:i32)
            n127 = Greater Or Equal To 0?(x=w491) -> (x >= 0?=w486:bool)
            n128 = Less?(x=w491, y=w471) -> (x < y?=w485:bool)
            n129 = Compound Arithmetic op=AND(w485, w486, w489) -> (w490:bool)
            n130 = case shown="True" w490 {
              selector: w490 -> [w495 _]
              tunnel: w488 -> [_ w500]
              tunnel: w484 -> [w494 w503]
              tunnel: [w492 w502] -> w483
              tunnel: [w495 w501] -> w478
              tunnel: w481 -> [w493 w498]
              tunnel: w474 -> [_ w499]
              tunnel: w479 -> [_ w497]
              tunnel: w477 -> [_ w496]
              frame False {
                n131 = call "ge_HideCellCtrls.vi"("error IO"=w494, "FP Ctrl"=w493) -> ("error out"=w492:errorcluster)  [unwired: 9 in]
              }
              frame True {
                n132 = call "ge_EditCell.vi"("Mod"=w497, "MeasType"=w499, "error in"=w503, "Active Cell"=w500, "ge_DAQManDefinitions"=w496, "FP Ctrl"=w498) -> ("error out"=w502:errorcluster, "Discard?"=w501:bool)  [unwired: 4 in]
              }
            }
          }
          frame "Ungchd Enter?" {
            n133 = property on="Property Node" class="MCListbox (strict)"(reference=w507, error in=w508) -> (error out=w519:errorcluster, "ItemNames"=w518:string[][], "ActiveCell"=w517:T8)  [unwired: 1 out]
            n134 = Unbundle By Name(w517) -> ("Row"=w520:i32, "Column"=w521:i32)
            n135 = Index Array(array=w518, index (row)=w520, index (col)=w521) -> (element=w522:string)
            n136 = property class="Ctl"(reference=w510, error in=w519) -> (reference out=w523:refnum<vi>, error out=w516:errorcluster, "Value"=w525:variant, "Label.Text"=w515:string)
            n137 = case shown="\"CellString\"" w515 {
              tunnel: w525 -> [_ w532 w537 w543]
              tunnel: [FALSE w531 w536 w542] -> w524
              tunnel: w522 -> [_ w528 w534 w539]
              frame Default {
              }
              frame "CellDbl" {
                n138 = Variant To Data(type=0.0, Variant=w532) -> (data=w530:dbl)  [unwired: 1 in, 1 out]
                n139 = Fract/Exp String To Number(string=w528) -> (number=w529:dbl)  [unwired: 3 in, 1 out]
                n140 = Equal?(x=w530, y=w529) -> (x = y?=w531:bool)
              }
              frame "CellString" {
                n141 = Variant To Data(type="", Variant=w537) -> (data=w535:string)  [unwired: 1 in, 1 out]
                n142 = Equal?(x=w535, y=w534) -> (x = y?=w536:bool)
              }
              frame "CellInt" {
                n143 = Variant To Data(type=0, Variant=w543) -> (data=w541:i32)  [unwired: 1 in, 1 out]
                n144 = Decimal String To Number(string=w539) -> (number=w540:i32)  [unwired: 2 in, 1 out]
                n145 = Equal?(x=w541, y=w540) -> (x = y?=w542:bool)
              }
            }
            n146 = case shown="True" w524 {
              tunnel: w523 -> [w544 w550]
              tunnel: w525 -> [_ w549]
              tunnel: w516 -> [w545 w548]
              tunnel: [w545 w547] -> w514
              tunnel: [w544 w546] -> w512
              frame False {
              }
              frame True {
                n147 = property class="Ctl"(reference=w550, error in=w548, "Val(Sgnl)"=w549) -> (reference out=w546:refnum<vi>, error out=w547:errorcluster)
              }
            }
            n148 = Close Reference(reference=w512, error in (no error)=w514) -> (error out=w513:errorcluster)
          }
          frame "Cell Key" {
            n149 = property class="ChanGrp.lvclass"(reference=w551, error in=w552) -> (error out=w554:errorcluster, "MeasType"=w553:T14)  [unwired: 1 out]
            n150 = property on="Property Node" class="MCListbox (strict)"(reference=w567, error in=w554) -> (error out=w562:errorcluster, "ItemNames"=w570:string[][], "ActiveCell"=w569:T8, "NumRows"=w556:u32, "TopLeft"=w557:T11)  [unwired: 1 out]
            n151 = property class="Ctl"(reference=w559, error in=w562, "Key Focus"=TRUE) -> (reference out=w563:refnum<vi>, error out=w564:errorcluster, "Value"=w561:variant, "Label.Text"=w560:string)
            n152 = case shown="\"Up\"..\"Right\"" w571 {
              selector: w571 -> [_ _ w656]
              tunnel: [w573 w585 w644] -> w572
              tunnel: w570 -> [_ w584 _]
              tunnel: w569 -> [_ w581 w650]
              tunnel: [FALSE FALSE TRUE] -> w568
              tunnel: w551 -> [_ _ w633]
              tunnel: w566 -> [_ _ w664]
              tunnel: w567 -> [_ _ w668]
              tunnel: w566 -> [_ w582 w662]
              tunnel: w564 -> [w573 w580 w660]
              tunnel: w563 -> [_ w579 _]
              tunnel: w561 -> [_ w578 _]
              tunnel: w560 -> [_ w577 w659]
              tunnel: w557 -> [_ _ w642]
              tunnel: w556 -> [_ _ w637]
              tunnel: w555 -> [_ w576 _]
              tunnel: w555 -> [_ _ w635]
              tunnel: w555 -> [_ _ w634]
              tunnel: w553 -> [_ w575 w632]
              frame Default {
              }
              frame "Enter", "Return" {
                # "I would like to have a value change event even\nif the user doesn't type anything new into the\ncontrol."
                # "The NumPad Enter key actually removes\nKeyFocus for booleans.  This call returns\nkey focus in case that happens."
                n153 = Unbundle By Name(w581) -> ("Row"=w586:i32, "Column"=w587:i32)
                n154 = Index Array(array=w584, index (row)=w586, index (col)=w587) -> (element=w588:string)
                n155 = case shown="\"CellHiLite\"" w577 {
                  tunnel: [w593 w599 w609 w617 w624] -> w590
                  tunnel: w580 -> [w593 w600 w608 w616 w623]
                  tunnel: w578 -> [_ _ w607 w615 w622]
                  tunnel: [FALSE FALSE w606 w614 w618] -> w589
                  tunnel: w588 -> [_ _ w603 w611 w619]
                  tunnel: w582 -> [_ w598 _ _ _]
                  tunnel: w581 -> [_ w597 _ _ _]
                  tunnel: w576 -> [_ w596 _ _ _]
                  tunnel: w575 -> [_ w595 _ _ _]
                  frame Default {
                  }
                  frame "CellHiLite" {
                    n156 = call "ge_EditCell.vi"("MeasType"=w595, "error in"=w600, "Active Cell"=w597, "ge_DAQManDefinitions"=w596, "FP Ctrl"=w598) -> ("error out"=w599:errorcluster)  [unwired: 5 in, 1 out]
                  }
                  frame "CellDbl" {
                    n157 = Fract/Exp String To Number(string=w603) -> (number=w604:dbl)  [unwired: 3 in, 1 out]
                    n158 = Variant To Data(error in=w608, type=0.0, Variant=w607) -> (data=w605:dbl, error out=w609:errorcluster)
                    n159 = Equal?(x=w604, y=w605) -> (x = y?=w606:bool)
                  }
                  frame "CellInt" {
                    n160 = Decimal String To Number(string=w611) -> (number=w612:i32)  [unwired: 2 in, 1 out]
                    n161 = Variant To Data(error in=w616, type=0, Variant=w615) -> (data=w613:i32, error out=w617:errorcluster)
                    n162 = Equal?(x=w612, y=w613) -> (x = y?=w614:bool)
                  }
                  frame "CellString" {
                    n163 = Variant To Data(error in=w623, type="", Variant=w622) -> (data=w621:string, error out=w624:errorcluster)
                    n164 = Equal?(x=w619, y=w621) -> (x = y?=w618:bool)
                  }
                }
                n165 = case shown="True" w589 {
                  tunnel: w579 -> [w626 w631]
                  tunnel: w578 -> [_ w630]
                  tunnel: w590 -> [w625 w629]
                  tunnel: [w626 w628] -> w591
                  tunnel: [w625 w627] -> w592
                  frame False {
                  }
                  frame True {
                    n166 = property class="Ctl"(reference=w631, error in=w629, "Val(Sgnl)"=w630) -> (reference out=w628:refnum<vi>, error out=w627:errorcluster)
                  }
                }
                n167 = Close Reference(reference=w591, error in (no error)=w592) -> (error out=w585:errorcluster)
              }
              frame "Up".."Right" {
                # "This logic is for situations when there are more rows\nthan are visible on table."
                n168 = call "ge_HideCellCtrls.vi"("error IO"=w660, "FP Ctrl"=w662) -> ("error out"=w646:errorcluster)  [unwired: 9 in]
                n169 = Not Equal?(x=w659, y="Pull Down") -> (x != y?=w657:bool)
                n170 = Unbundle By Name(w650) -> ("Row"=w667:i32, "Column"=w666:i32)
                n171 = Select(t=w656, s=w657, f=eventvkey."ASCII") -> (s? t:f=w655:T1)
                n172 = Unbundle By Name(w642) -> ("Row"=w638:u32)
                n173 = case shown="\"Down\"" w655 {
                  tunnel: [w676 w678 w691 w700 w704] -> w639
                  tunnel: w667 -> [w676 w681 w692 w700 w704]
                  tunnel: [w675 w682 w693 w698 w702] -> w665
                  tunnel: w666 -> [w675 w682 w693 w699 w703]
                  tunnel: w638 -> [w674 w677 w687 w697 w701]
                  tunnel: w637 -> [_ _ w689 _ _]
                  tunnel: [w674 w680 w686 w697 w701] -> w636
                  frame Default {
                  }
                  frame "Up" {
                    n174 = Decrement(x=w681) -> (x-1=w678:i32)
                    n175 = Less?(x=w678, y=w677) -> (x < y?=w679:bool)
                    n176 = case shown="True" w679 {
                      tunnel: w677 -> [w683 w685]
                      tunnel: [w683 w684] -> w680
                      frame False {
                      }
                      frame True {
                        n177 = Decrement(x=w685) -> (x-1=w684:u32)
                      }
                    }
                  }
                  frame "Down" {
                    n178 = Increment(x=w692) -> (x+1=w691:i32)
                    n179 = Subtract(x=w691, y=w687) -> (x-y=w690:u32)
                    n180 = Greater Or Equal?(x=w690, y=w689) -> (x >= y?=w688:bool)
                    n181 = case shown="True" w688 {
                      tunnel: w687 -> [w694 w696]
                      tunnel: [w694 w695] -> w686
                      frame False {
                      }
                      frame True {
                        n182 = Increment(x=w696) -> (x+1=w695:u32)
                      }
                    }
                  }
                  frame "Left" {
                    n183 = Decrement(x=w699) -> (x-1=w698:i32)
                  }
                  frame "Right" {
                    n184 = Increment(x=w703) -> (x+1=w702:i32)
                  }
                }
                n185 = Bundle By Name(cluster=w650, "Row"=w639, "Column"=w665) -> (w651:T8)
                n186 = Bundle By Name(cluster=w642, "Row"=w636) -> (w641:T11)
                n187 = Unbundle By Name(w651) -> ("Row"=w669:i32, "Column"=w649:i32)
                n188 = call "GetChanContents.vi"("ChanGrp.lvclass"=w633) -> ("Num of Chans"=w672:i32)  [unwired: 4 in, 6 out]
                n189 = call "ge_NumInputCols.vi"("MeasType"=w632, "ge_DAQManDefinitions"=w635) -> ("Max Input Col"=w647:i32)  [unwired: 7 in]
                n190 = Greater Or Equal To 0?(x=w669) -> (x >= 0?=w670:bool)
                n191 = Greater?(x=w649, y=2) -> (0:w652:bool)
                n192 = Less?(x=w649, y=w647) -> (x < y?=w648:bool)
                n193 = Less?(x=w669, y=w672) -> (x < y?=w671:bool)
                n194 = Compound Arithmetic op=AND(w671, w670, w652, w648) -> (invert w640:bool)
                n195 = Select(t=w650, s=w640, f=w651) -> (s? t:f=w663:T8)
                n196 = Select(t=w642, s=w640, f=w641) -> (s? t:f=w643:T11)
                n197 = property class="MCListbox (strict)"(reference=w668, error in=w646, "ActiveCell"=w663, "TopLeft"=w643) -> (error out=w645:errorcluster)  [unwired: 1 out]
                n198 = call "ge_EditCell.vi"("HiLite"=TRUE ("PD HiLite"), "MeasType"=w632, "error in"=w645, "Active Cell"=w663, "ge_DAQManDefinitions"=w634, "FP Ctrl"=w664) -> ("error out"=w644:errorcluster)  [unwired: 4 in, 1 out]
              }
            }
          }
          frame "Cell ValChng" {
            n199 = case shown="Default" w707 {
              tunnel: w714 -> [_ w734]
              tunnel: w713 -> [w715 w718]
              tunnel: w705 -> [_ w719]
              tunnel: w711 -> [_ w732]
              tunnel: w710 -> [_ w731]
              tunnel: [w715 w728] -> w709
              tunnel: w706 -> [_ w720]
              frame "Up".."Right" {
                # "This disables the feature where LabVIEW will increment, decrement a value when you press up or down."
              }
              frame Default {
                n200 = property class="ChanGrp.lvclass"(reference=w719, error in=w718) -> (error out=w717:errorcluster, "MeasType"=w716:T14)  [unwired: 1 out]
                n201 = property class="Ctl"(reference=w734, error in=w717) -> (reference out=w737:refnum<vi>, error out=w736:errorcluster, "Label.Text"=w730:string, "Value"=w733:variant)
                n202 = call "ge_FindFPCtrl.vi"("Ctrl Name"=w730, "FP Ctrl"=w731) -> ("Ctrl Ref"=w729:refnum<vi>)  [unwired: 3 in]
                n203 = Close Reference(reference=w737, error in (no error)=w736) -> (error out=w735:errorcluster)
                n204 = call "CellColors.vi"() -> ("Normal"=w738:u32)  [unwired: 8 in, 3 out]
                n205 = case shown="\"Pull Down\"" w730 {
                  tunnel: [w743 w747 w771 w782 w790] -> w739
                  tunnel: w735 -> [w743 w749 w778 w788 w798]
                  tunnel: [w742 w746 w776 w786 w794] -> w722
                  tunnel: ["" ("String") w745 w775 w780 w795] -> w723
                  tunnel: w738 -> [w742 _ w776 w786 w794]
                  tunnel: w733 -> [_ w748 w774 w785 w793]
                  tunnel: w729 -> [_ w744 w770 w781 w789]
                  frame Default {
                  }
                  frame "Pull Down" {
                    n206 = Variant To Data(error in=w749, type=u16 0, Variant=w748) -> (data=w758:u16, error out=w750:errorcluster)
                    n207 = To More Specific Class(target class=refnum<vi> refnum ("reference"), reference=w744, error in=w750) -> (specific class reference=w752:refnum<vi>, error out=w751:errorcluster)
                    n208 = property on="Property Node" class="Ring (strict)"(reference=w752, error in=w751, "Value"=u16 65535, "HideLastVal"=TRUE ("Hide Last Value"), "Visible"=FALSE) -> (error out=w747:errorcluster, "StringsAndValues[]"=w756:T22)  [unwired: 1 out]
                    n209 = for {
                      tunnel: w756 -> [w769] mode=indexing
                      tunnel: [w768] -> w759 mode=indexing
                      n210 = Unbundle By Name(w769) -> ("Value"=w768:u16)
                    }
                    n211 = Array Size(array=w756) -> (size(s)=w767:i32)
                    n212 = Less Or Equal?(x=w767, y=2) -> (x <= y?=w765:bool)
                    n213 = call "CellColors.vi"() -> ("Disabled"=w764:u32, "Normal"=w763:u32)  [unwired: 8 in, 2 out]
                    n214 = Search 1D Array(1D array=w759, element=w758) -> (index of element=w757:i32)  [unwired: 1 in]
                    n215 = Index Array(array=w756, index=w757) -> (element=w755:cluster{"String":string, "Value":u16})
                    n216 = Select(t=w764, s=w765, f=w763) -> (s? t:f=w746:u32)
                    n217 = Unbundle By Name(w755) -> ("String"=w745:string)
                  }
                  frame "CellString" {
                    n218 = Variant To Data(error in=w778, type="", Variant=w774) -> (data=w775:string, error out=w772:errorcluster)
                    n219 = property on="Property Node" class="Ctl"(reference=w770, error in=w772, "Visible"=FALSE) -> (error out=w771:errorcluster)  [unwired: 1 out]
                  }
                  frame "CellDbl" {
                    n220 = Variant To Data(error in=w788, type=0.0, Variant=w785) -> (data=w779:dbl, error out=w783:errorcluster)
                    n221 = call "StringCnvPrecision.vi"("Number"=w779) -> ("Float String"=w780:string)  [unwired: 6 in]
                    n222 = property on="Property Node" class="Ctl"(reference=w781, error in=w783, "Visible"=FALSE) -> (error out=w782:errorcluster)  [unwired: 1 out]
                  }
                  frame "CellInt" {
                    n223 = Variant To Data(error in=w798, type=0, Variant=w793) -> (data=w796:i32, error out=w791:errorcluster)
                    n224 = Number To Decimal String(number=w796) -> (decimal integer string=w795:string)  [unwired: 1 in]
                    n225 = property on="Property Node" class="Ctl"(reference=w789, error in=w791, "Visible"=FALSE) -> (error out=w790:errorcluster)  [unwired: 1 out]
                  }
                }
                n226 = property on="Property Node" class="MCListbox (strict)"(reference=w732, error in=w739) -> (reference out=w740:refnum<vi>, error out=w725:errorcluster, "ItemNames"=w727:string[][], "ActiveCell"=w721:T8)
                n227 = call "ge_CellIndicators.vi"("MeasType"=w716, "ge_DAQManDefinitions"=w720, "error in"=w725, "Cell Contents"=w723, "ActiveCell"=w721, "Item Names"=w727) -> ("error out"=w724:errorcluster, "Item Names"=w726:string[][])  [unwired: 4 in]
                n228 = property on="Property Node" class="MCListbox (strict)"(reference=w740, error in=w724, "ItemNames"=w726, "CellBG"=w722) -> (error out=w728:errorcluster)  [unwired: 1 out]
              }
            }
          }
          frame "Click Ring" {
            w807 = T17 {"Hdr Width"=120, "Glbl Ctrl"=enum."Ring0"}  # HdrInfo
            # "Table def for meas type"
            # "Returns all support for all ring ctrls for all active channels"
            # "Get name of the ring ctrl that was clicked"
            # "Get supported Ring values for all selected rows"
            # "Get all Glbl Ctrls for this Measurement Type"
            n229 = To More Specific Class(target class=refnum<vi> refnum ("reference"), reference=w830, error in=w820) -> (specific class reference=w826:refnum<vi>, error out=w825:errorcluster)
            n230 = property class="ChanGrp.lvclass"(reference=w799) -> ("MeasType"=w800:T14)  [unwired: 1 in, 2 out]
            n231 = call "ge_SelRows.vi"("error in"=w820, "ChanGrp.lvclass"=w799, "Table Ref"=w832) -> ("error out"=w821:errorcluster, "Selected Rows"=w822:i32[])  [unwired: 7 in]
            n232 = property class="Ring (strict)"(reference=w826, error in=w825) -> (reference out=w823:refnum<vi>, error out=w814:errorcluster, "Label.Text"=w811:string)
            n233 = call "ge_PopGlobals.vi"("error in"=w821, "Selected Rows"=w822, "ChanGrp.lvclass"=w799, "ge_DAQManDefinitions"=w802) -> ("error out"=w819:errorcluster, "DefVal"=w804:u16, "Ring Support For Group"=w818:variant)  [unwired: 5 in]
            n234 = Unbundle By Name(w802) -> ("Table Definitions"=w801:variant)
            n235 = Format Into String(error in=w814, w800) -> (resulting string=w816:string, error out=w817:errorcluster)  [unwired: 2 in]
            n236 = Get Variant Attribute(Variant=w801, name=w816, default value (empty Variant)=variant ("All Ring Support"), error in=w817) -> (value=w812:variant, error out=w813:errorcluster)  [unwired: 2 out]
            n237 = Get Variant Attribute(Variant=w812, error in=w813) -> (duplicate Variant=w809:variant, names=w806:string[], error out=w810:errorcluster)  [unwired: 2 in, 1 out]
            n238 = for {
              tunnel: w806 -> [w859] mode=indexing
              tunnel: w809 -> [w861]
              shift-right: [w856] -> w805
              shift-left: w810 -> [w860]
              tunnel: [w854] -> w808 mode=indexing
              tunnel: w807 -> [w853]
              n239 = Get Variant Attribute(Variant=w861, name=w859, default value (empty Variant)=w853, error in=w860) -> (value=w858:T17, error out=w857:errorcluster)  [unwired: 2 out]
              n240 = Unbundle By Name(w858) -> ("Glbl Ctrl"=w855:T10)
              n241 = Format Into String(error in=w857, w855) -> (resulting string=w854:string, error out=w856:errorcluster)  [unwired: 2 in]
            }
            n242 = Search 1D Array(1D array=w808, element=w811) -> (index of element=w803:i32)  [unwired: 1 in]
            n243 = case shown="Default" w803 {
              selector: w803 -> [_ w836]
              tunnel: [w835 w852] -> w829
              tunnel: [u16 0 ("Value") w851] -> w827
              tunnel: w823 -> [_ w850]
              tunnel: w819 -> [w835 w846]
              tunnel: w818 -> [_ w845]
              tunnel: w806 -> [_ w844]
              tunnel: w805 -> [_ w842]
              tunnel: w804 -> [_ w837]
              frame -1 {
              }
              frame Default {
                n244 = Index Array(array=w844, index=w836) -> (element=w843:string)
                n245 = Get Variant Attribute(Variant=w845, name=w843, default value (empty Variant)=T9[] [] ("String and Values"), error in=w846) -> (value=w839:T9[], error out=w841:errorcluster)  [unwired: 2 out]
                n246 = Merge Errors(w841, w842) -> (w840:errorcluster)
                n247 = property on="Property Node" class="Ring (strict)"(reference=w850, error in=w840, "StringsAndValues[]"=w839, "Value"=w837) -> (reference out=w848:refnum<vi>, error out=w849:errorcluster)
                n248 = Index Array(array=w839) -> (element=w838:T9)  [unwired: 1 in]
                n249 = Unbundle By Name(w838) -> ("Value"=w851:u16)
                n250 = Close Reference(reference=w848, error in (no error)=w849) -> (error out=w852:errorcluster)
              }
            }
            "ValIfDismissed" <- w827
          }
          frame "Dismiss Menu" {
            w875 = FALSE ("Visible")
            n251 = call "ge_FindFPCtrl.vi"("Ctrl Name"="Pull Down" ("Name"), "FP Ctrl"=w865) -> ("Ctrl Ref"=w866:refnum<vi>)  [unwired: 3 in]
            n252 = To More Specific Class(target class=refnum<vi> refnum ("reference"), reference=w866, error in=w867) -> (specific class reference=w869:refnum<vi>, error out=w868:errorcluster)
            n253 = property on="Property Node" class="Ring (strict)"(reference=w869, error in=w868, "Visible"=w875, "Key Focus"=w875) -> (error out=w874:errorcluster)  [unwired: 1 out]
          }
          frame "Glbl Apply" {
            n254 = property class="ChanGrp.lvclass"(reference=w880, error in=w878) -> (reference out=w876:refnum<class "ChanGrp.lvclass">, error out=w877:errorcluster, "MeasType"=w879:T14)
            n255 = property class="Ctl"(reference=w898, error in=w877) -> (reference out=w896:refnum<vi>, error out=w897:errorcluster, "Label.Text"=w886:string)
            n256 = Match Pattern(string=w886, regular expression="[0-9]+") -> (before substring=w890:string)  [unwired: 1 in, 3 out]
            n257 = call "ge_GetHdrInfo.vi"("ge_DAQManDefinitions"=w885, "MeasType"=w879) -> ("Glbl Ctrls"=w884:T10[], "Hdr Name"=w883:T16[])  [unwired: 7 in, 1 out]
            n258 = case shown="\"Cal\"" w890 {
              tunnel: w896 -> [w915 w922]
              tunnel: w897 -> [w917 w921]
              tunnel: [w917 w920] -> w895
              tunnel: [w915 w919] -> w893
              tunnel: [variant ("Value") w918] -> w892
              frame "Cal" {
              }
              frame Default {
                n259 = property class="Ctl"(reference=w922, error in=w921) -> (reference out=w919:refnum<vi>, error out=w920:errorcluster, "Value"=w918:variant)
              }
            }
            n260 = for {
              tunnel: w884 -> [w912] mode=indexing
              tunnel: [w911] -> w881 mode=indexing
              n261 = Format Into String(w912) -> (resulting string=w911:string)  [unwired: 3 in, 1 out]
            }
            n262 = Close Reference(reference=w893, error in (no error)=w895) -> (error out=w894:errorcluster)
            n263 = for {
              tunnel: w883 -> [w914] mode=indexing
              tunnel: [w913] -> w882 mode=indexing
              n264 = Format Into String(w914) -> (resulting string=w913:string)  [unwired: 3 in, 1 out]
            }
            n265 = property on="Property Node" class="MCListbox (strict)"(reference=w889, error in=w894) -> (reference out=w907:refnum<vi>, error out=w910:errorcluster, "ItemNames"=w902:string[][])
            n266 = call "ge_SelRows.vi"("error in"=w910, "ChanGrp.lvclass"=w876, "Table Ref"=w907) -> ("error out"=w903:errorcluster, "Selected Rows"=w904:i32[])  [unwired: 7 in]
            n267 = Search 1D Array(1D array=w881, element=w886) -> (index of element=w899:i32)  [unwired: 1 in]
            n268 = call "GetGrp Devices.vi"("Selected Rows"=w904, "ChanGrp.lvclass"=w876) -> ("Dev Array"=w908:string[])  [unwired: 8 in, 1 out]
            n269 = Index Array(array=w882, index=w899) -> (element=w888:string)
            n270 = for {
              shift-right: [w934] -> w906
              shift-left: w903 -> [w938]
              tunnel: w904 -> [w927] mode=indexing
              tunnel: w908 -> [w933] mode=indexing
              shift-right: [w935] -> w905
              shift-left: w902 -> [w936]
              tunnel: w886 -> [w931]
              tunnel: w892 -> [w930]
              tunnel: w889 -> [w929]
              tunnel: w879 -> [w928]
              tunnel: w879 -> [w926]
              tunnel: w888 -> [w925]
              tunnel: w885 -> [w924]
              tunnel: w885 -> [w923]
              stop <- w934 stop-if-true
              n271 = call "ge_GetGlblString.vi"("Value"=w930, "ge_DAQManDefinitions"=w923, "Label.Text"=w931, "MeasType"=w926, "error in"=w938, "Row"=w927, "Header"=w925, "Device"=w933) -> ("error out"=w937:errorcluster, "Cell Contents"=w932:T5[])  [unwired: 2 in]
              n272 = for {
                shift-right: [w942] -> w934
                shift-left: w937 -> [w941]
                shift-right: [w947] -> w935
                shift-left: w936 -> [w944]
                tunnel: w932 -> [w949] mode=indexing
                tunnel: w929 -> [w948]
                tunnel: w928 -> [w946]
                tunnel: w927 -> [_]
                tunnel: w924 -> [w939]
                n273 = Unbundle By Name(w949) -> ("Coords"=w945:T6, "Cell Contents.Cell BG Color"=w950:u32, "Cell Contents.Cell Text"=w943:string)
                n274 = call "ge_CellIndicators.vi"("MeasType"=w946, "ge_DAQManDefinitions"=w939, "error in"=w941, "Cell Contents"=w943, "ActiveCell"=w945, "Item Names"=w944) -> ("error out"=w940:errorcluster, "Item Names"=w947:string[][])  [unwired: 4 in]
                n275 = property on="Property Node" class="MCListbox (strict)"(reference=w948, error in=w940, "ActiveCell"=w945, "CellBG"=w950) -> (error out=w942:errorcluster)  [unwired: 1 out]
              }
            }
            n276 = property on="Property Node" class="MCListbox (strict)"(reference=w889, error in=w906, "ItemNames"=w905) -> (error out=w900:errorcluster)  [unwired: 1 out]
          }
          frame "Calibrate" {
            n277 = property class="Ctl"(reference=w961, error in=w962) -> (reference out=w965:refnum<vi>, error out=w964:errorcluster, "Label.Text"=w960:string)
            n278 = Close Reference(reference=w965, error in (no error)=w964) -> (error out=w963:errorcluster)
            n279 = property class="ChanGrp.lvclass"(reference=w952) -> ("MeasType"=w951:T14)  [unwired: 1 in, 2 out]
            n280 = call "ge_SelRows.vi"("error in"=w963, "ChanGrp.lvclass"=w952, "Table Ref"=w954) -> ("error out"=w956:errorcluster, "Selected Rows"=w969:i32[])  [unwired: 7 in]
            n281 = property on="Property Node" class="MCListbox (strict)"(reference=w954, error in=w956) -> (reference out=w958:refnum<vi>, error out=w957:errorcluster, "ItemNames"=w955:string[][])
            n282 = Unbundle By Name(w968) -> ("Group Specific Info.Chassis Name"=w967:string)
            n283 = case shown="\"Voltage\", \"Strain\"" w951 {
              selector: w951 -> [_ w974 _]
              tunnel: w969 -> [_ w982 w1019]
              tunnel: w967 -> [_ w981 w1018]
              tunnel: [w971 w980 w1016] -> w966
              tunnel: w960 -> [_ w979 _]
              tunnel: w951 -> [_ w978 w1013]
              tunnel: w958 -> [_ w977 _]
              tunnel: w957 -> [w971 w976 w1020]
              tunnel: w955 -> [_ w975 w1015]
              tunnel: w954 -> [_ _ w1014]
              tunnel: w953 -> [_ w973 w1010]
              tunnel: w953 -> [_ w972 w1011]
              frame Default {
              }
              frame "Voltage", "Strain" {
                n284 = for {
                  shift-right: [w996] -> w980
                  shift-left: w976 -> [w988]
                  tunnel: w982 -> [w993] mode=indexing
                  tunnel: w981 -> [w995]
                  tunnel: w979 -> [w991]
                  tunnel: w977 -> [w989]
                  tunnel: w978 -> [w990]
                  tunnel: w974 -> [w986]
                  shift-right: [w985] -> _
                  shift-left: w975 -> [w987]
                  tunnel: w973 -> [w984]
                  tunnel: w972 -> [w983]
                  stop <- w996 stop-if-true
                  n285 = Index Array(array=w987, index (row)=w993) -> (element=w992:string[])  [unwired: 1 in]
                  n286 = call "ge_CalibrateSingleChan.vi"("Chassis Name"=w995, "Ctrl Name"=w991, "MeasType"=w986, "error in"=w988, "Row"=w993, "ItemNames"=w992, "ge_DAQManDefinitions"=w984) -> ("error out"=w997:errorcluster, "Cell Contents"=w994:T5[])  [unwired: 3 in]
                  n287 = for {
                    shift-right: [w1008] -> w996
                    shift-left: w997 -> [w1001]
                    tunnel: w994 -> [w1007] mode=indexing
                    shift-right: [w1004] -> w985
                    shift-left: w987 -> [w1005]
                    tunnel: w989 -> [w1006]
                    tunnel: w990 -> [w999]
                    tunnel: w983 -> [w998]
                    n288 = Unbundle By Name(w1007) -> ("Coords"=w1003:T6, "Cell Contents.Cell BG Color"=w1009:u32, "Cell Contents.Cell Text"=w1002:string)
                    n289 = call "ge_CellIndicators.vi"("MeasType"=w999, "ge_DAQManDefinitions"=w998, "error in"=w1001, "Cell Contents"=w1002, "ActiveCell"=w1003, "Item Names"=w1005) -> ("error out"=w1000:errorcluster, "Item Names"=w1004:string[][])  [unwired: 4 in]
                    n290 = property on="Property Node" class="MCListbox (strict)"(reference=w1006, error in=w1000, "ActiveCell"=w1003, "CellBG"=w1009, "ItemNames"=w1004) -> (error out=w1008:errorcluster)  [unwired: 1 out]
                  }
                }
              }
              frame "Dynamic" {
                n291 = call "ge_CalibrateDynamic.vi"("Chassis Name"=w1018, "Selected Rows"=w1019, "error in"=w1020, "ge_DAQManDefinitions"=w1010, "ItemNames"=w1015) -> ("error out"=w1017:errorcluster, "Cell Contents"=w1012:T5[])  [unwired: 5 in]
                n292 = for {
                  shift-right: [w1031] -> w1016
                  shift-left: w1017 -> [w1024]
                  tunnel: w1012 -> [w1030] mode=indexing
                  shift-right: [w1027] -> _
                  shift-left: w1015 -> [w1028]
                  tunnel: w1014 -> [w1029]
                  tunnel: w1013 -> [w1022]
                  tunnel: w1011 -> [w1021]
                  n293 = Unbundle By Name(w1030) -> ("Coords"=w1026:T6, "Cell Contents.Cell BG Color"=w1032:u32, "Cell Contents.Cell Text"=w1025:string)
                  n294 = call "ge_CellIndicators.vi"("MeasType"=w1022, "ge_DAQManDefinitions"=w1021, "error in"=w1024, "Cell Contents"=w1025, "ActiveCell"=w1026, "Item Names"=w1028) -> ("error out"=w1023:errorcluster, "Item Names"=w1027:string[][])  [unwired: 4 in]
                  n295 = property on="Property Node" class="MCListbox (strict)"(reference=w1029, error in=w1023, "ActiveCell"=w1026, "CellBG"=w1032, "ItemNames"=w1027) -> (error out=w1031:errorcluster)  [unwired: 1 out]
                }
              }
            }
          }
          frame "Apply Settings" {
            n296 = property class="MCListbox (strict)"(reference=w1041, error in=w1034) -> (error out=w1033:errorcluster, "ItemNames"=w1038:string[][])  [unwired: 1 out]
            n297 = call "ConvertTbl2ChanGrp.vi"("error in (no error)"=w1033, "ItemNames"=w1038, "ge_DAQManDefinitions"=w1037, "ChanGrp in"=w1036) -> ("error out"=w1039:errorcluster, "ChanGrp in"=w1035:refnum<class "ChanGrp.lvclass">)  [unwired: 6 in]
          }
          frame "Shutdown" {
            n298 = Unbundle By Name(w1053) -> ("This VI"=w1052:refnum<vi>)
            n299 = invoke class="VI" method="FP.Close"(reference=w1052, error in=w1055) -> (reference out=w1049:refnum<vi>, error out=w1050:errorcluster)  [unwired: 1 in, 1 out]
            n300 = Close Reference(reference=w1049, error in (no error)=w1050) -> (error out=w1048:errorcluster)
            n301 = call "ge_ClearBoneyard.vi"("error in"=w1048, "FP Ctrl"=w1047) -> ("error out"=w1046:errorcluster)  [unwired: 9 in]
            "ChanGrp.lvclass" <- w1044
          }
        }
      }
    }
    frame Error {
    }
  }
  "error out" <- w11
  "Discard?" <- w3
